vi "Mean ex Inf.vi"(9 "Array":dbl[](array[numeric])) -> (1 "Mean ex Inf":dbl format="%0.2f")   [LabVIEW 2019]
uses:
  <vilib>/Analysis/baseanly.llb/Mean (DBL).vi
  <vilib>/Analysis/NI_AALBase.lvlib
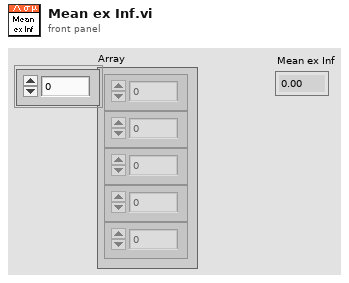
[diagram p1: front panel]
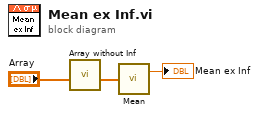
[diagram p0: block diagram]
diagram:
  n1 = call "Array without Inf.vi"("Input Array"="Array") -> ("Array without Inf"=w2:dbl[])  [unwired: 10 in]
  n2 = call-poly <vilib>:"Mean.vi"("X"=w2) -> ("mean"=→"Mean ex Inf":dbl)  [unwired: 1 out]
